vi "OvershootProtection.vi"(1 "Log fO2 rel. IW/IM":dbl, 2 "Set Point (*C)":dbl) -> (0 "Overshoot protection":dbl)   [LabVIEW 2009]
uses:
  <vilib>/gmath/interp.llb/Interpolate 2D (2d X,Y).vi
  <vilib>/gmath/NI_Gmath.lvlib
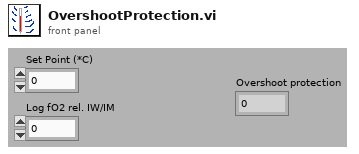
[diagram p1: front panel]
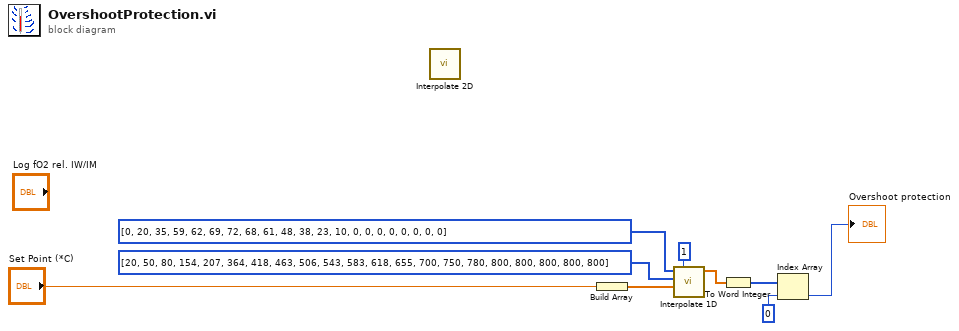
[diagram p0: block diagram]
diagram:
  n1 = call-poly <vilib>:"Interpolate 2D.vi"() -> ()  [unwired: 8 in, 4 out]
  n2 = Build Array("Set Point (*C)") -> (w8:dbl[])
  n3 = call <vilib>:"Interpolate 1D.vi"("method"=1, "xi"=w8, "X"=i32[] [20, 50, 80, 154, 207, 364, 418, 463, 506, 543, 583, 618, 655, 700, 750, 780, 800, 800, 800, 800, 800], "Y"=i32[] [0, 20, 35, 59, 62, 69, 72, 68, 61, 48, 38, 23, 10, 0, 0, 0, 0, 0, 0, 0, 0]) -> ("yi"=w6:dbl[])  [unwired: 5 in, 2 out]
  n4 = To Word Integer(number=w6) -> (16bit integer=w5:i16[])
  n5 = Index Array(array=w5, index=0) -> (element=→"Overshoot protection":i16)
